vi "kepcoScan.vi"   [LabVIEW 2014]
uses:
  <vilib>/Platform/TimedLoop/XDataNode/timing_clust.ctl
  <vilib>/Platform/TimedLoop/XDataNode/nitl_modes.ctl
  <vilib>/Platform/TimedLoop/XDataNode/wakeup.ctl
  <vilib>/rvi/Emulation/niFpgaGetClockAttributes.vi
  <vilib>/rvi/Emulation/niFpgaSctlEmulationGetInTimedLoop.vi
  <vilib>/rvi/Emulation/niFpgaEmulationReportErrorSimple.vi
  <vilib>/rvi/Emulation/niFpgaCriticalErrorInLSC.vi
  <vilib>/rvi/Emulation/niFpgaEmulationIsFPGAContextNoSignature.vi
  <vilib>/rvi/DataTransferAndStorage/Container/Common/niFpgaContainerGetUniqueNameForEmu.vi
  <vilib>/rvi/eio/common/nirviEmuReportErrorAndStop.vi
  <vilib>/rvi/Emulation/niFpgaProcessEmulError.vi
  DAC/Code/FPGA SPI_Globals.vi
  <vilib>/rvi/eio/common/nirviEmuTemplateMethod_errors.vi
  <vilib>/Platform/TimedLoop/XDataNode/XDataNode.xnode
  <vilib>/rvi/DataTransferAndStorage/Container/XNode/niFpgaContainer.xnode
  <vilib>/rvi/DataTransferAndStorage/Handshake/Emulation/niFpgaHandshakeEmulation.vi
  <vilib>/eio/EIONode/EIONode.xnode
  <vilib>/Platform/TimedLoop/XDataNode/XDNodeRunTimeDep.lvlib
types:
  T1 = typedef "XDNodeRunTimeDep.lvlib/timing_clust.ctl" = cluster{"Expected End [f-1]":u64, "Actual End [f-1]":u64, "Finished Late? [f-1]":bool, "Expected End [i-1]":u64, "Actual End [i-1]":u64, "Finished Late? [i-1]":bool, "Expected Start [i]":u64, "Actual Start [i]":u64, "Expected Start [f]":u64, "Actual Start [f]":u64, "Source Name":string, "Structure Name":string, "Period":i64, "Deadline":i64, "Offset":i64, "Start":i64, "Priority":i32, "Timeout":i32, "Mode":T2, "Wakeup Reason":T3, "Error":errorcluster, "Source Type":string, "Secondary Source Type":string, "Global End Time":u64, "Global Start Time":u64, "Frame Duration":u64, "Iteration Duration":u64, "Assigned CPU":i32, "I/O Scan Engine Mode":u32}
  T2 = typedef "XDNodeRunTimeDep.lvlib/nitl_modes.ctl" = enum32{"No Change", "Process missed periods, maintain original phase", "Discard missed periods, maintain original phase", "Process missed periods, ignore original phase", "Discard missed periods, ignore original phase"}
  T3 = typedef "XDNodeRunTimeDep.lvlib/wakeup.ctl" = enum32{"Normal", "Aborted", "Asynchronous wakeup", "Timing source error", "Timed loop error", "Timeout"}
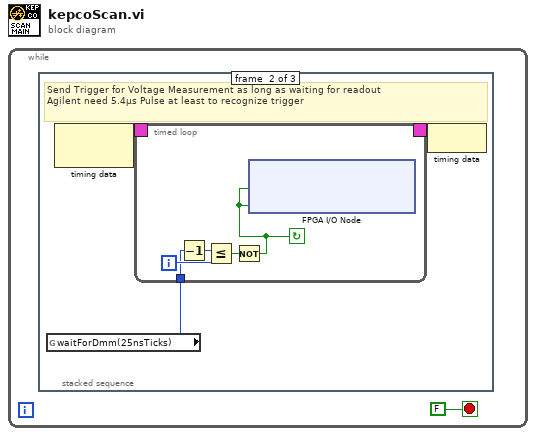
[diagram p0: block diagram]
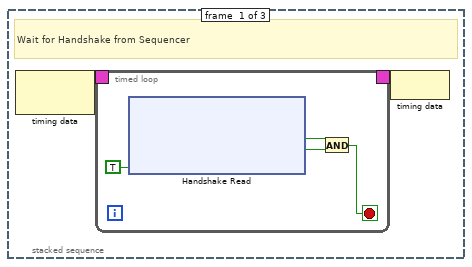
[diagram p2: hidden frame]
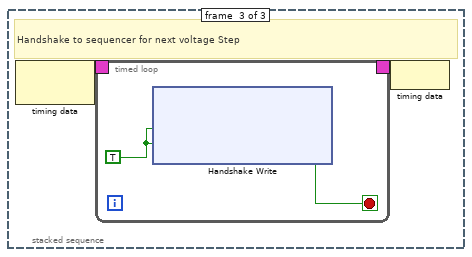
[diagram p3: hidden frame]
diagram:
  n1 = while {
    stop <- FALSE stop-if-true
    n2 = stacked-sequence {
      frame #0 {
        # "Wait for Handshake from Sequencer"
        n3 = node-c288() -> (w3:T1)  [unwired: 1 in]
        n4 = timed-loop {
          timing: w3 -> [_]
          timing-out: [_] -> w2
          stop <- w4 stop-if-true
          n5 = xnode ("Handshake Read")("Ready for Output"=TRUE) -> ("Data"=w6:bool, "Output Valid"=w5:bool)  [unwired: 1 in, 1 out]
          n6 = And(x=w6, y=w5) -> (x .and. y?=w4:bool)
        }
        n7 = node-c288(w2) -> ()
      }
      frame #1 {
        # "Send Trigger for Voltage Measurement as long as waiting for readout\nAgilent need 5.4µs Pulse at least to recognize trigger"
        n8 = global read "FPGA SPI_Globals.vi" "waitForDmm(25nsTicks)"() -> (w12:i32)
        n9 = node-c288() -> (w14:T1)  [unwired: 1 in]
        n10 = timed-loop {
          timing: w14 -> [_]
          timing-out: [_] -> w13
          tunnel: w12 -> [w18]
          i -> [w19]
          stop <- w15 continue-if-true
          n11 = Decrement(x=w18) -> (x-1=w17:i32)
          n12 = Less Or Equal?(x=w17, y=w19) -> (x <= y?=w16:bool)
          n13 = Not(x=w16) -> (.not. x?=w15:bool)
          n14 = xnode "FPGA I/O Node"("PXI_Trig3"=w15, "measVoltFlagDio8Con1"=w15) -> ()  [unwired: 2 in, 2 out]
        }
        n15 = node-c288(w13) -> ()
      }
      frame #2 {
        # "Handshake to sequencer for next voltage Step"
        n16 = node-c288() -> (w25:T1)  [unwired: 1 in]
        n17 = timed-loop {
          timing: w25 -> [_]
          timing-out: [_] -> w24
          stop <- w27 stop-if-true
          w26 = TRUE ("Ready for Output")
          n18 = xnode ("Handshake Write")("Data"=w26, "Input Valid"=w26) -> ("Ready for Input"=w27:bool)  [unwired: 1 in, 1 out]
        }
        n19 = node-c288(w24) -> ()
      }
    }
  }
